vi "Custom Automation Tool.vi"(8 "error in (no error)":errorcluster) -> (0 "error out":errorcluster)   [LabVIEW 2021]
doc: "Presents an interface to either update a specification limit, or add a new one."
uses:
  CTLs/Step.ctl
  CTLs/Step Type.ctl
  <vilib>/Utility/config.llb/Config Data RefNum.ctl
  <vilib>/Utility/miscctls.llb/LVRowAndColumnUnsignedTypeDef.ctl
  CTLs/FGV Actions.ctl
  bd503c13-d10c-440e-ab5e-4e60baef5deb.vi
  cc7d3372-ed48-481f-8659-91fce09351ce.vi
  <vilib>/Utility/config.llb/Write Key (String).vi
  <vilib>/Utility/config.llb/Read Key (String).vi
  <userlib>/_MGI/Application Control/MGI Gray if/MGI Gray if False.vi
  <vilib>/Utility/inputDevices.llb/closeKeyboard.vi
  <vilib>/Utility/inputDevices.llb/keyboardAcquire.vi
  <vilib>/Utility/config.llb/NI_LVConfig.lvlib
  FaKI State Machine/FaKI State Machine.lvlib
panel:
  in  "Export":bool
  in  "Import":bool
  out "Application Hotkey":string
  in  "Delete":bool
  in  "Start/Stop":bool
  in  "N":i32 caption="Times to Repeat\n(-1 = indefinitely)" min=-1
  in  "Activation Type":enum32{"Hotkey", "Automatic"}(radio)
  out "Menu":bool
  out "Row":i32
  in  "Add Step 2":bool
  in  "Dbl Click":T1
  out "Table":string[][](table)
  in  "Clear Profile":bool
  in  "Delete Step":bool
  in  "Insert Step":bool
  in  "Add Step":bool
  in  "Modify Step":bool
  in  "Close":bool
  in  "Save":bool
  in  "Restore":bool
  in  "Help":bool
  in  "Process Name":string(combo)
  # "Table has double-click\nfunctionality"
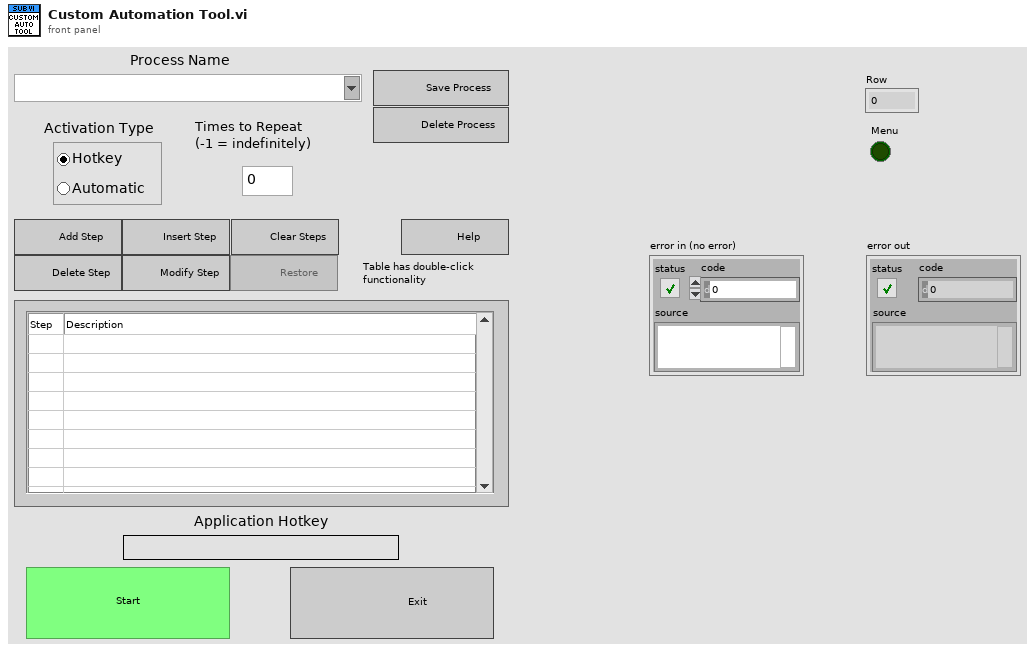
[diagram p1: front panel]
types:
  T1 = cluster{"Insert Before":bool, "Insert After":bool, "Modify":bool, "Delete":bool}
  T2 = enum8{"Enabled", "Disabled", "Disabled and Grayed Out"}
  T3 = typedef "LVPoint32TypeDef.ctl" = cluster{"Horizontal":i32, "Vertical":i32}
  T4 = typedef "LVRowAndColumnTypeDef.ctl" = cluster{"Row":i32, "Column":i32}
  T5 = enum32{"Invalid", "Standard", "Closed", "Hidden", "Minimized", "Maximized"}
  T6 = enum32{"invalid app kind", "Development System", "Run Time System", "Student Edition", "Embedded LabVIEW", "Evaluation", "Custom"}
  T7 = typedef "Step.ctl" = cluster{"Type":T8, "Coords":cluster{"x":i32, "y":i32}, "Delay":i32, "Key":u8, "Repeat":i32, "RClick?":bool}
  T8 = typedef "Step Type.ctl" = enum16{"Mouse Move", "Mouse Click", "Key Press", "Wait", "Mouse Down", "Mouse Up", "Key Down", "Key Up"}
  T9 = typedef "LVRowAndColumnUnsignedTypeDef.ctl" = cluster{"Row":u32, "Column":u32}
  T10 = cluster{"Steps":T7[], "Activation Type":enum32{"Hotkey", "Automatic"}, "N":i32}
  T11 = typedef "FGV Actions.ctl" = enum16{"Read", "Write"}
  T12 = typedef "NI_LVConfig.lvlib/Config Data RefNum.ctl" = refnum<k1>
  T13 = cluster{"Core":cluster{"Current VI Reference":refnum<vi>, "Close Panel on Exit?":bool}, "Steps":T7[], "Refs":refnum<vi>[], "Config":T12, "Step":i32, "n":i32, "Hotkey":enum16{"0", "1", "2", "3", "4", "5", "6", "7", "8", "9", "A", "B", "C", "D", "E", "F", "G", "H", "I", "J", "K", "L", "M", "N", "O", "P", "Q", "R", "S", "T", "U", "V", "W", "X", "Y", "Z", "F1", "F2", "F3", "F4", "F5", "F6", "F7", "F8", "F9", "F10", "F11", "F12", "F13", "F14", "F15", "ADD", "BACK", "BACKSLASH", "CAPITAL", "COMMA", "DECIMAL", "DELETE", "DIVIDE", "DOWN", "END", "EQUALS", "ESCAPE", "GRAVE (`)", "HOME", "INSERT", "LBRACKET", "LCONTROL", "LEFT", "L ALT", "LSHIFT", "LWIN", "MINUS", "MULTIPLY", "NEXT", "NUMLOCK", "NUMPAD_0", "NUMPAD_1", "NUMPAD_2", "NUMPAD_3", "NUMPAD_4", "NUMPAD_5", "NUMPAD_6", "NUMPAD_7", "NUMPAD_8", "NUMPAD_9", "PAUSE", "PERIOD", "PRIOR (PG UP)", "RBRACKET", "RCONTROL", "RETURN", "RIGHT", "R ALT", "RSHIFT", "RWIN", "SCROLL", "SEMICOLON", "SLASH", "SPACE", "SUBTRACT", "TAB", "UP", "ENTER (num pad)", "' (quote)"}[], "Keyboard":refnum<k1>}
  T14 = enum16{"0", "1", "2", "3", "4", "5", "6", "7", "8", "9", "A", "B", "C", "D", "E", "F", "G", "H", "I", "J", "K", "L", "M", "N", "O", "P", "Q", "R", "S", "T", "U", "V", "W", "X", "Y", "Z", "F1", "F2", "F3", "F4", "F5", "F6", "F7", "F8", "F9", "F10", "F11", "F12", "F13", "F14", "F15", "ADD", "BACK", "BACKSLASH", "CAPITAL", "COMMA", "DECIMAL", "DELETE", "DIVIDE", "DOWN", "END", "EQUALS", "ESCAPE", "GRAVE (`)", "HOME", "INSERT", "LBRACKET", "LCONTROL", "LEFT", "L ALT", "LSHIFT", "LWIN", "MINUS", "MULTIPLY", "NEXT", "NUMLOCK", "NUMPAD_0", "NUMPAD_1", "NUMPAD_2", "NUMPAD_3", "NUMPAD_4", "NUMPAD_5", "NUMPAD_6", "NUMPAD_7", "NUMPAD_8", "NUMPAD_9", "PAUSE", "PERIOD", "PRIOR (PG UP)", "RBRACKET", "RCONTROL", "RETURN", "RIGHT", "R ALT", "RSHIFT", "RWIN", "SCROLL", "SEMICOLON", "SLASH", "SPACE", "SUBTRACT", "TAB", "UP", "ENTER (num pad)", "' (quote)"}[]
  T15 = cluster{"Current VI Reference":refnum<vi>, "Close Panel on Exit?":bool}
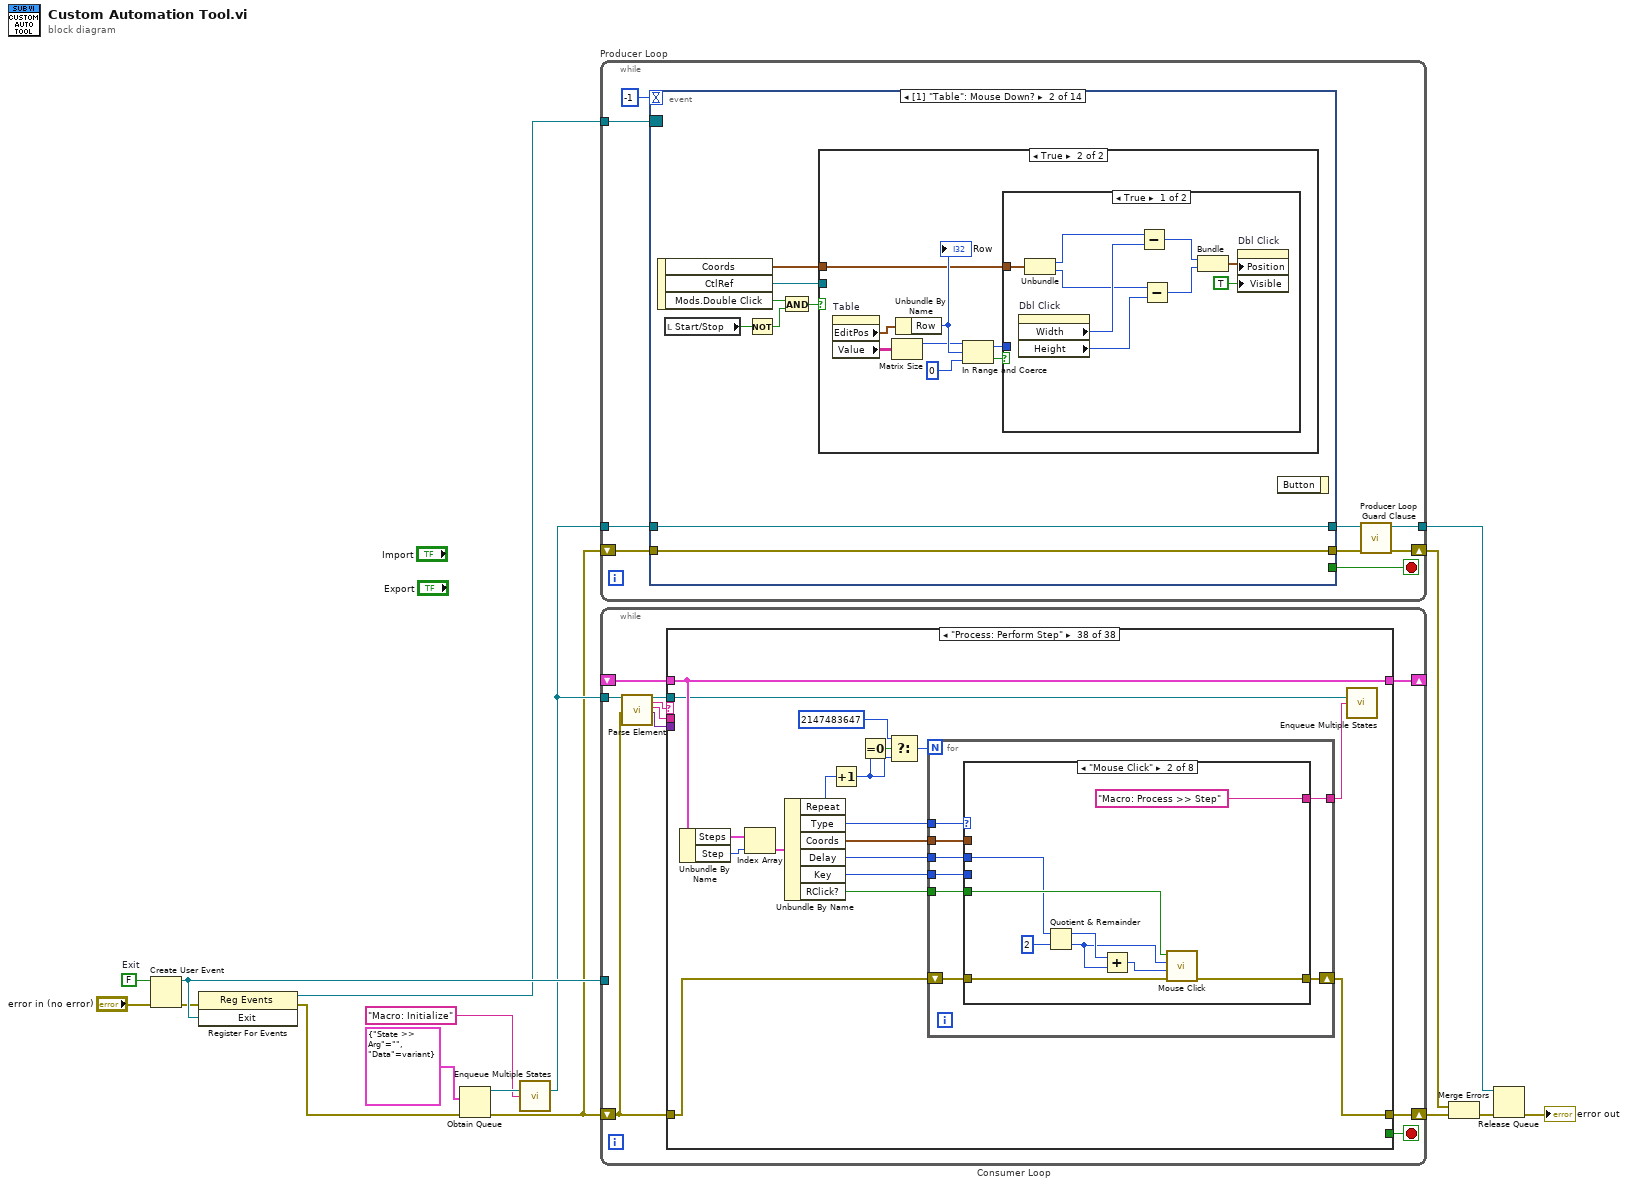
[diagram p0: block diagram]
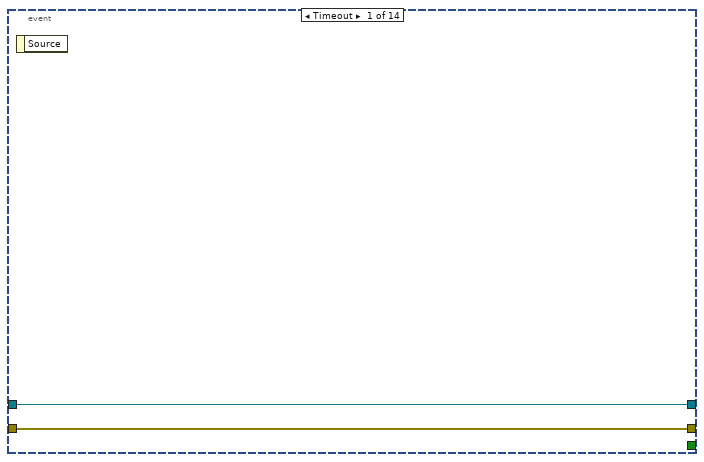
[diagram p2: hidden frame]
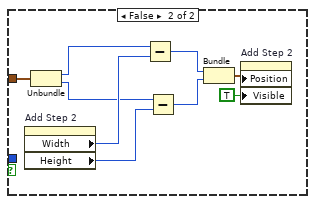
[diagram p4: hidden frame]
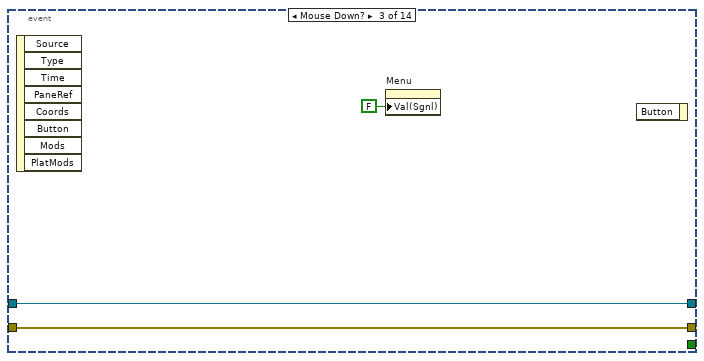
[diagram p5: hidden frame]
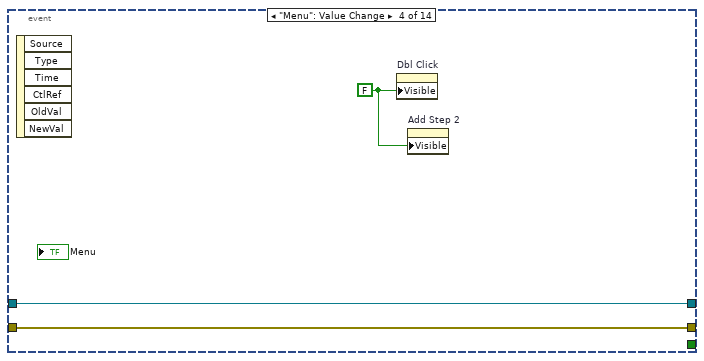
[diagram p6: hidden frame]
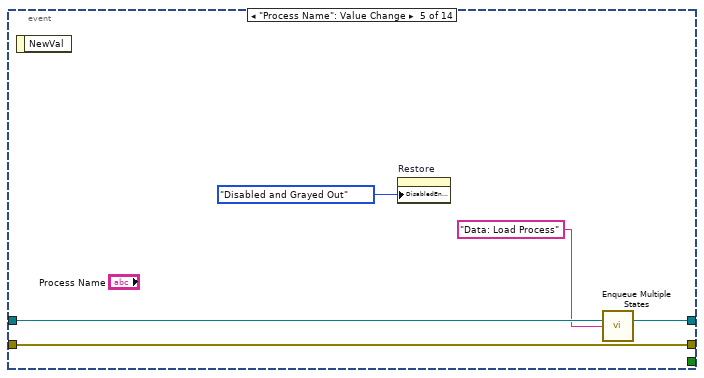
[diagram p7: hidden frame]
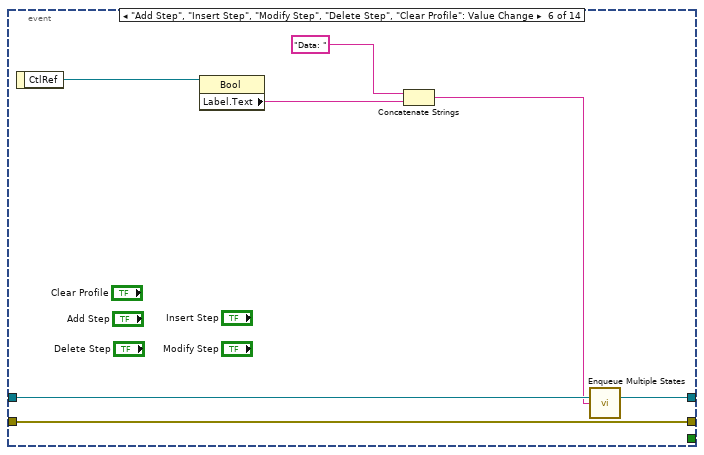
[diagram p8: hidden frame]
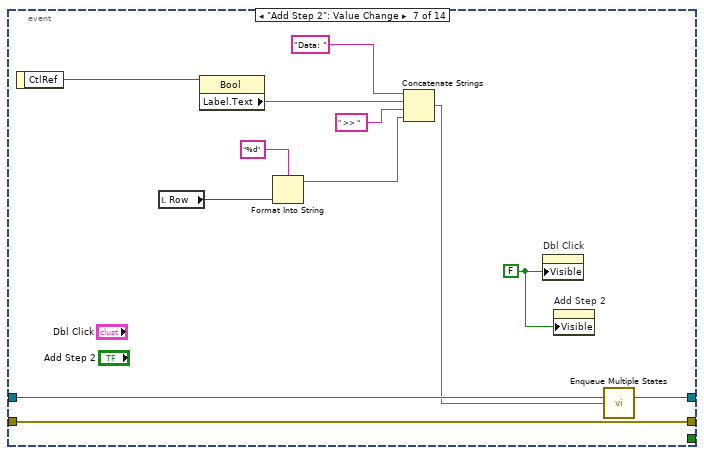
[diagram p9: hidden frame]
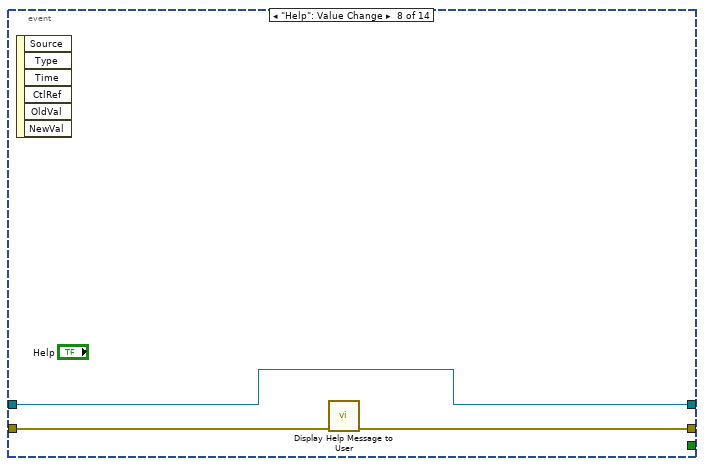
[diagram p10: hidden frame]
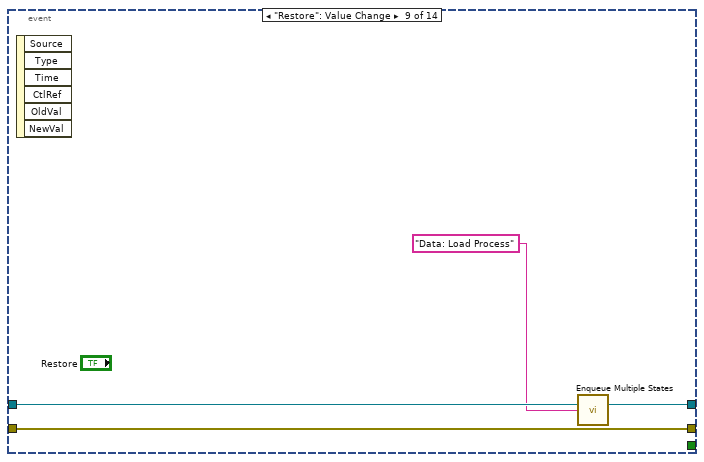
[diagram p11: hidden frame]
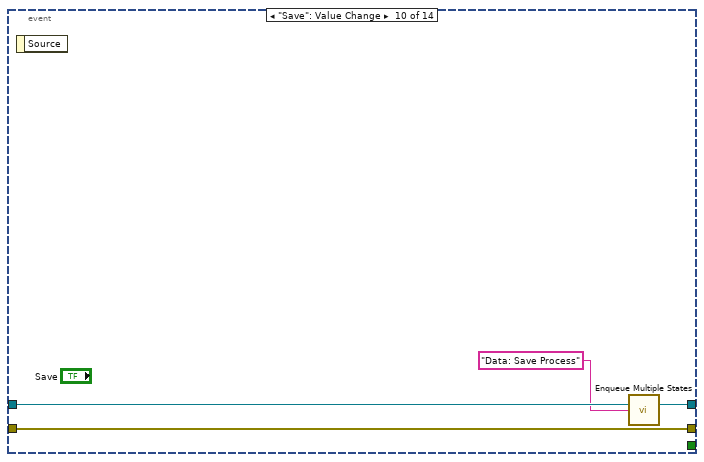
[diagram p12: hidden frame]
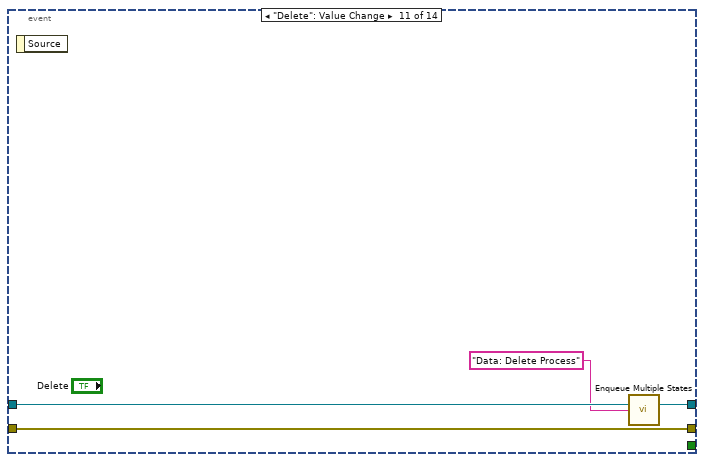
[diagram p13: hidden frame]
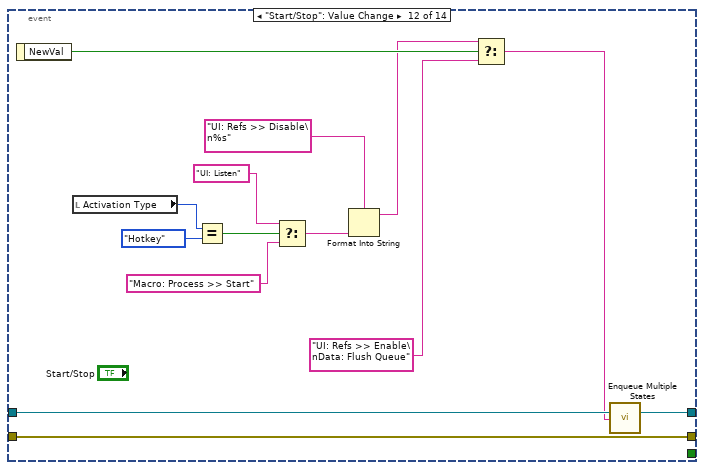
[diagram p14: hidden frame]
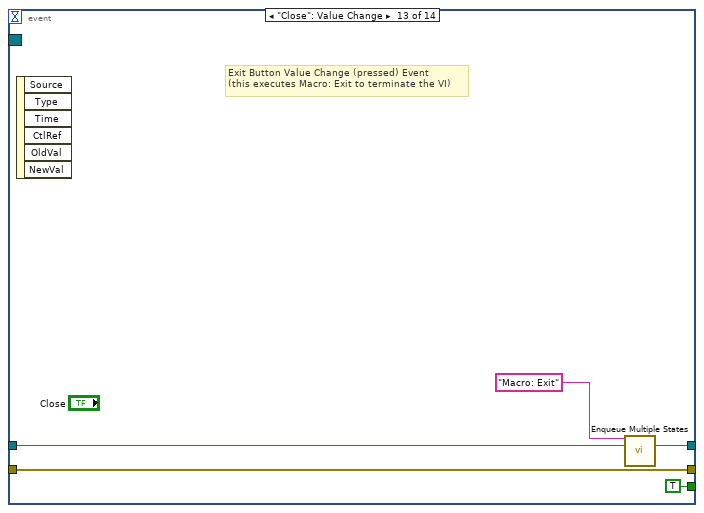
[diagram p15: hidden frame]
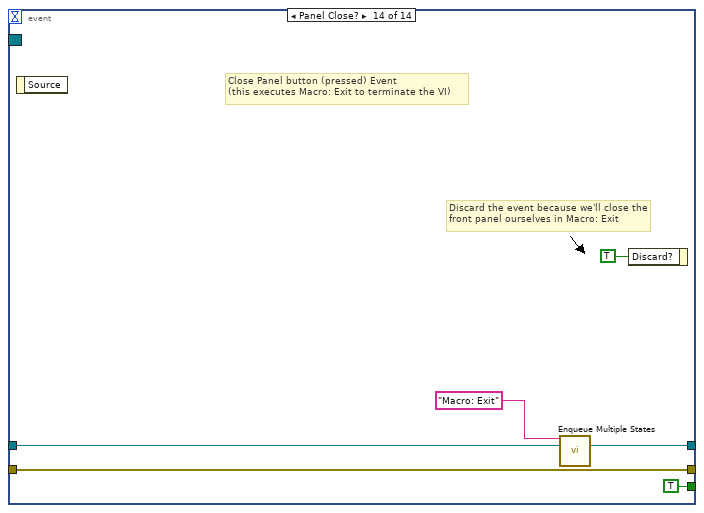
[diagram p16: hidden frame]
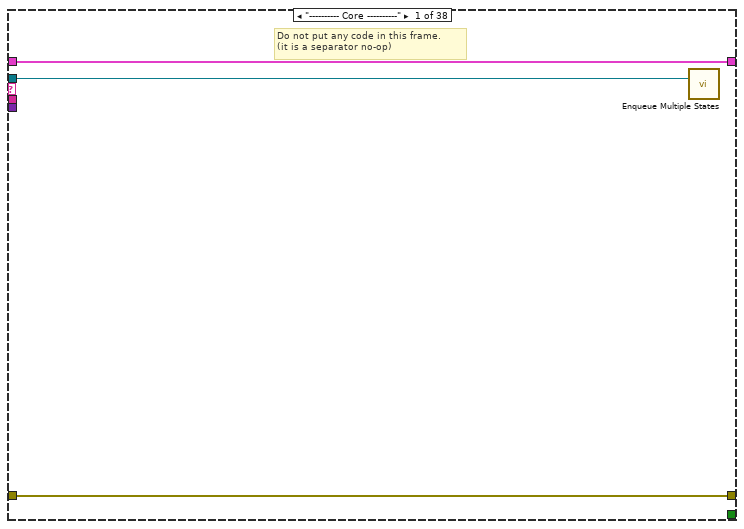
[diagram p17: hidden frame]
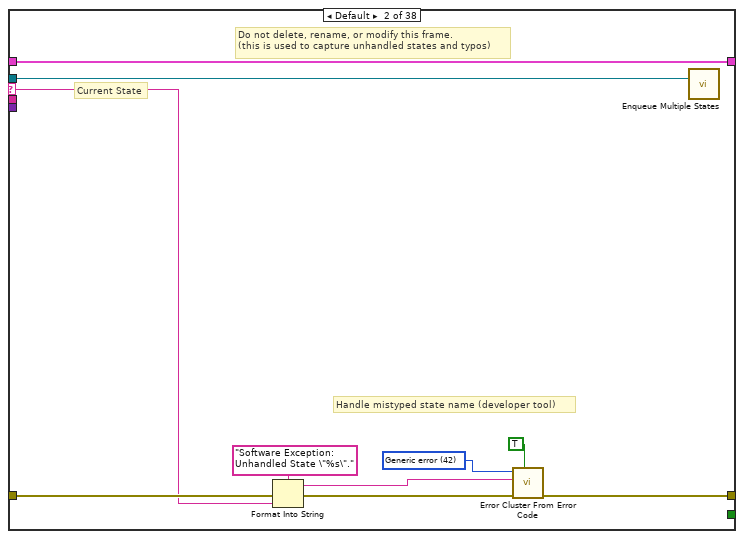
[diagram p18: hidden frame]
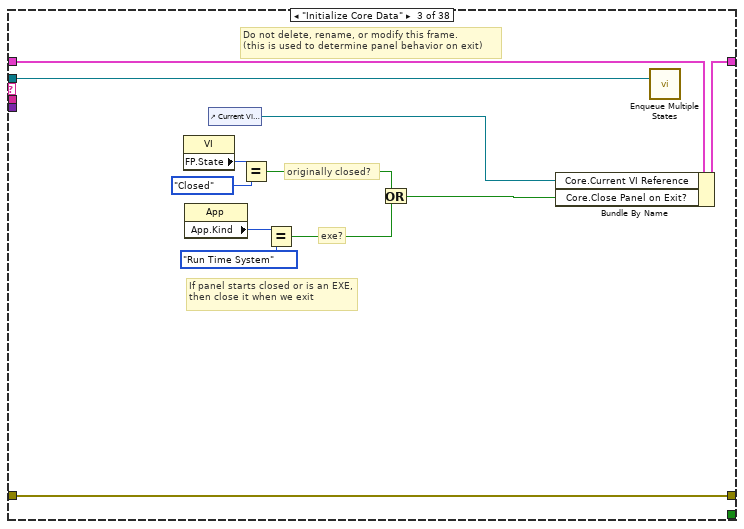
[diagram p19: hidden frame]
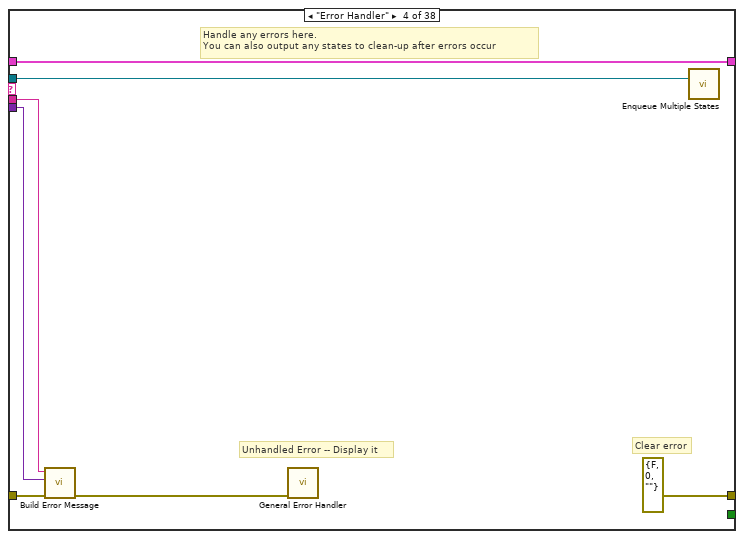
[diagram p20: hidden frame]
diagram:
  w13 = FALSE  # Exit
  n1 = Create User Event(user event datatype=w13, error in="error in (no error)") -> (user event=w16:refnum<user-event>, error out=w12:errorcluster)
  n2 = register-events(error in=w12, w16) -> (reference out=w15:refnum<event-registration>, error out=w14:errorcluster)  [unwired: 1 in]
  n3 = Obtain Queue(element data type=cluster{"State >> Arg":string, "Data":variant} {"State >> Arg"="", "Data"=variant}, error in (no error)=w14) -> (queue out=w6:refnum<queue>, error out=w3:errorcluster)  [unwired: 3 in, 1 out]
  n4 = call "Enqueue Multiple States.vi"("queue in"=w6, "State(s) at Back"="Macro: Initialize") -> ("queue out"=w7:refnum<queue>)  [unwired: 13 in]
  n5 = while "Producer Loop" {
    shift-right: [w25] -> w9
    shift-left: w3 -> [w23]
    tunnel: w15 -> [w19]
    tunnel: w7 -> [w21]
    tunnel: [w24] -> w11
    stop <- w18 stop-if-true
    n6 = event shown="[1] \"Table\": Mouse Down?" {
      selector: w19 -> [_ _ _ _ _ _ _ _ _ _ _ _ _ _]
      dyn-events: _ -> [_ _ _ _ _ _ _ _ _ _ _ _ _ _]
      timeout: -1 ("Timeout") -> [_ _ _ _ _ _ _ _ _ _ _ _ _ _]
      tunnel: [w27 w35 w64 w67 w72 w79 w91 w93 w98 w102 w106 w120 w125 w131] -> w22
      tunnel: w23 -> [w27 w35 w64 w67 w72 w79 w91 w94 w98 w102 w106 w120 w125 w131]
      tunnel: w21 -> [w26 w32 w62 w65 w70 w75 w82 w92 w96 w101 w105 w108 w123 w128]
      tunnel: [w26 w32 w62 w65 w69 w74 w81 w92 w97 w100 w104 w109 w122 w127] -> w20
      tunnel: [_ _ _ _ _ _ _ _ _ _ _ _ TRUE TRUE] -> w18
      event Timeout {
        n7 = event-data() -> ()  [unwired: 1 in, 1 out]
      }
      event "Table": Mouse Down? {
        n8 = event-data() -> ("Coords"=w33:T3, "CtlRef"=w34:refnum<vi>, "Mods.Double Click"=w29:bool)  [unwired: 1 in]
        n9 = local read "Start/Stop"() -> (w31:bool)
        n10 = Not(x=w31) -> (.not. x?=w30:bool)
        n11 = And(x=w29, y=w30) -> (x .and. y?=w28:bool)
        n12 = case shown="True" w28 {
          tunnel: w34 -> [_ _]
          tunnel: w33 -> [_ w36]
          frame False {
          }
          frame True {
            n13 = property on="Table" class="Tbl (strict)"() -> ("EditPos"=w42:T4, "Value"=w43:string[][])  [unwired: 2 in, 2 out]
            n14 = Matrix Size(0:w43) -> (1:w40:i32)  [unwired: 1 out]
            n15 = Unbundle By Name(w42) -> ("Row"=w41:i32)
            "Row" <- w41
            n16 = In Range and Coerce(upper limit=w40, x=w41, lower limit=0) -> (coerced(x)=w37:i32, In Range?=w38:bool)
            n17 = case shown="True" w38 {
              tunnel: w37 -> [_ _]
              tunnel: w36 -> [w51 w60]
              frame True {
                n18 = property on="Dbl Click" class="Clust"() -> ("Width"=w49:u32, "Height"=w48:u32)  [unwired: 2 in, 2 out]
                n19 = Unbundle(w51) -> ("Horizontal"=w50:i32, "Vertical"=w47:i32)
                n20 = Subtract(x=w50, y=w49) -> (x-y=w45:u32)
                n21 = Subtract(x=w47, y=w48) -> (x-y=w46:u32)
                n22 = Bundle(w45, w46) -> (w44:cluster{u32, u32})  [unwired: 1 in]
                n23 = property on="Dbl Click" class="Clust"("Position"=w44, "Visible"=TRUE) -> ()  [unwired: 2 in, 2 out]
              }
              frame False {
                n24 = property on="Add Step 2" class="Bool"() -> ("Width"=w58:u32, "Height"=w57:u32)  [unwired: 2 in, 2 out]
                n25 = Unbundle(w60) -> ("Horizontal"=w59:i32, "Vertical"=w56:i32)
                n26 = Subtract(x=w59, y=w58) -> (x-y=w54:u32)
                n27 = Subtract(x=w56, y=w57) -> (x-y=w55:u32)
                n28 = Bundle(w54, w55) -> (w53:cluster{u32, u32})  [unwired: 1 in]
                n29 = property on="Add Step 2" class="Bool"("Position"=w53, "Visible"=TRUE) -> ()  [unwired: 2 in, 2 out]
              }
            }
          }
        }
        n30 = event-data() -> ()  [unwired: 2 in, 1 out]
      }
      event Mouse Down? {
        n31 = event-data() -> ()  [unwired: 1 in, 8 out]
        n32 = property on="Menu" class="Bool (strict)"("Val(Sgnl)"=FALSE ("Value (Signaling)")) -> ()  [unwired: 2 in, 2 out]
        n33 = event-data() -> ()  [unwired: 2 in, 1 out]
      }
      event "Menu": Value Change {
        w66 = FALSE ("Visible")
        n34 = event-data() -> ()  [unwired: 1 in, 6 out]
        n35 = property on="Dbl Click" class="Clust"("Visible"=w66) -> ()  [unwired: 2 in, 2 out]
        n36 = property on="Add Step 2" class="Bool"("Visible"=w66) -> ()  [unwired: 2 in, 2 out]
      }
      event "Process Name": Value Change {
        n37 = event-data() -> ()  [unwired: 1 in, 1 out]
        n38 = property on="Restore" class="Bool"("DisabledEnum"=T2."Disabled and Grayed Out" ("Disabled")) -> ()  [unwired: 2 in, 2 out]
        n39 = call "Enqueue Multiple States.vi"("queue in"=w70, "State(s) at Back"="Data: Load Process" ("string")) -> ("queue out"=w69:refnum<queue>)  [unwired: 13 in]
      }
      event "Add Step", "Insert Step", "Modify Step", "Delete Step", "Clear Profile": Value Change {
        n40 = event-data() -> ("CtlRef"=w78:refnum<vi>)  [unwired: 1 in]
        n41 = property class="Bool"(reference=w78) -> ("Label.Text"=w76:string)  [unwired: 1 in, 2 out]
        n42 = Concatenate Strings("Data: " ("State(s) at Back (\"\")"), w76) -> (w73:string)
        n43 = call "Enqueue Multiple States.vi"("queue in"=w75, "State(s) at Back"=w73) -> ("queue out"=w74:refnum<queue>)  [unwired: 13 in]
      }
      event "Dbl Click.Insert Before", "Dbl Click.Insert After", "Dbl Click.Modify", "Dbl Click.Delete", "Add Step 2": Value Change {
        w84 = FALSE ("Visible")
        n44 = event-data() -> ("CtlRef"=w90:refnum<vi>)  [unwired: 1 in]
        n45 = local read "Row"() -> (w83:i32)
        n46 = property class="Bool"(reference=w90) -> ("Label.Text"=w88:string)  [unwired: 1 in, 2 out]
        n47 = Format Into String(format string="%d", w83) -> (resulting string=w85:string)  [unwired: 2 in, 1 out]
        n48 = Concatenate Strings("Data: " ("State(s) at Back (\"\")"), w88, " >> " ("string"), w85) -> (w80:string)
        n49 = property on="Dbl Click" class="Clust"("Visible"=w84) -> ()  [unwired: 2 in, 2 out]
        n50 = property on="Add Step 2" class="Bool"("Visible"=w84) -> ()  [unwired: 2 in, 2 out]
        n51 = call "Enqueue Multiple States.vi"("queue in"=w82, "State(s) at Back"=w80) -> ("queue out"=w81:refnum<queue>)  [unwired: 13 in]
      }
      event "Help": Value Change {
        n52 = event-data() -> ()  [unwired: 1 in, 6 out]
        n53 = call "Display Help Message to User"("error in (no error)"=w94) -> ("error out"=w93:errorcluster)  [unwired: 9 in, 1 out]
      }
      event "Restore": Value Change {
        n54 = event-data() -> ()  [unwired: 1 in, 6 out]
        n55 = call "Enqueue Multiple States.vi"("queue in"=w96, "State(s) at Back"="Data: Load Process" ("State(s) at Back (\"\")")) -> ("queue out"=w97:refnum<queue>)  [unwired: 13 in]
      }
      event "Save": Value Change {
        n56 = event-data() -> ()  [unwired: 1 in, 1 out]
        n57 = call "Enqueue Multiple States.vi"("queue in"=w101, "State(s) at Back"="Data: Save Process" ("State(s) at Back (\"\")")) -> ("queue out"=w100:refnum<queue>)  [unwired: 13 in]
      }
      event "Delete": Value Change {
        n58 = event-data() -> ()  [unwired: 1 in, 1 out]
        n59 = call "Enqueue Multiple States.vi"("queue in"=w105, "State(s) at Back"="Data: Delete Process" ("State(s) at Back (\"\")")) -> ("queue out"=w104:refnum<queue>)  [unwired: 13 in]
      }
      event "Start/Stop": Value Change {
        n60 = event-data() -> ("NewVal"=w112:bool)  [unwired: 1 in]
        n61 = local read "Activation Type"() -> (w119:enum32{"Hotkey", "Automatic"})
        n62 = Equal?(x=w119, y=enum32{"Hotkey", "Automatic"}."Hotkey") -> (x = y?=w117:bool)
        n63 = Select(t="UI: Listen", s=w117, f="Macro: Process >> Start") -> (s? t:f=w114:string)
        n64 = Format Into String(format string="UI: Refs >> Disable\n%s" ("State(s) at Back (\"\")"), w114) -> (resulting string=w111:string)  [unwired: 2 in, 1 out]
        n65 = Select(t=w111, s=w112, f="UI: Refs >> Enable\nData: Flush Queue") -> (s? t:f=w107:string)
        n66 = call "Enqueue Multiple States.vi"("queue in"=w108, "State(s) at Back"=w107) -> ("queue out"=w109:refnum<queue>)  [unwired: 13 in]
      }
      event "Close": Value Change {
        # "Exit Button Value Change (pressed) Event\n(this executes Macro: Exit to terminate the VI)"
        n67 = event-data() -> ()  [unwired: 1 in, 6 out]
        n68 = call "Enqueue Multiple States.vi"("State(s) at Front"="Macro: Exit", "queue in"=w123) -> ("queue out"=w122:refnum<queue>)  [unwired: 13 in]
      }
      event Panel Close? {
        # "Discard the event because we'll close the front panel ourselves in Macro: Exit"
        # "Close Panel button (pressed) Event\n(this executes Macro: Exit to terminate the VI)"
        n69 = event-data() -> ()  [unwired: 1 in, 1 out]
        n70 = call "Enqueue Multiple States.vi"("State(s) at Front"="Macro: Exit", "queue in"=w128) -> ("queue out"=w127:refnum<queue>)  [unwired: 13 in]
        n71 = event-data("Discard?"=TRUE) -> ()  [unwired: 1 in, 1 out]
      }
    }
    n72 = call "Producer Loop Guard Clause.vi"("error in (no error)"=w22, "queue in"=w20) -> ("error out"=w25:errorcluster, "queue out"=w24:refnum<queue>)  [unwired: 8 in]
  }
  n73 = while "Consumer Loop" {
    shift-right: [w136] -> _
    shift-left: _ -> [w137]
    shift-right: [w139] -> w8
    shift-left: w3 -> [w140]
    tunnel: w7 -> [w141]
    tunnel: w16 -> [_]
    stop <- w138 stop-if-true
    n74 = call "Parse Element.vi"("queue in"=w141, "error in (no error)"=w140) -> ("queue out"=w135:refnum<queue>, "State"=w134:string, "Arg"=w133:string, "Data"=w132:variant)  [unwired: 14 in]
    n75 = case shown="\"Process: Perform Step\"" w134 {
      selector: w134 -> [_ w146 _ _ _ _ _ _ _ _ _ _ _ _ _ _ _ _ _ _ _ _ _ _ _ _ _ _ _ _ _ _ _ _ _ _ _ _]
      tunnel: w135 -> [w142 w145 w155 w167 w174 w178 w184 w207 _ w217 w225 w233 w241 w249 w257 w268 w280 w291 w302 _ w354 _ w396 w401 w410 w412 w421 _ w497 _ w522 w532 w545 w548 w553 w597 w604 w608]
      tunnel: w133 -> [_ _ _ w169 _ _ _ _ _ _ _ _ _ _ w259 w271 w282 w293 _ _ _ _ _ _ _ w413 w422 _ _ w515 _ _ _ _ w556 _ _ _]
      tunnel: w137 -> [w143 w148 w161 w172 w177 w179 _ w208 w212 w220 w226 w234 w242 w250 w260 w272 w283 w294 w304 w314 w351 w380 w400 w402 w406 w416 w424 w496 w510 w514 w530 w535 w546 w550 w552 w602 w605 w624]
      tunnel: [w144 w150 w165 errorcluster {"status"=FALSE, "code"=0, "source"=""} ("error out") w176 w180 w186 w209 w213 w221 w229 w237 w245 w253 w263 w275 w286 w297 w307 w321 w360 w381 w398 w403 w408 w414 w425 w494 w507 w513 w529 w536 w547 w551 w557 w603 w606 w615] -> w139
      tunnel: w140 -> [w144 w149 w165 w171 w176 w180 w187 w209 w214 w221 w229 w237 w245 w253 w263 w275 w286 w297 w307 w323 w365 w382 w397 w403 w409 w415 w426 w495 w508 w513 w526 w537 w547 w551 w557 w603 w606 w616]
      tunnel: [_ _ _ _ TRUE _ _ _ _ _ _ _ _ _ _ _ _ _ _ _ _ _ _ _ _ _ _ _ _ _ _ _ _ _ _ _ _ _] -> w138
      tunnel: [w143 w148 w166 w172 w177 w179 w206 w208 w211 w219 w228 w236 w244 w252 w262 w274 w285 w296 w303 w320 w352 w380 w400 w402 w405 w416 w424 w496 w510 w514 w530 w535 w546 w550 w555 w602 w605 w624] -> w136
      tunnel: w132 -> [_ _ _ w168 _ _ _ _ _ _ _ _ _ _ _ _ _ _ _ _ _ _ _ _ _ _ _ _ _ _ _ _ _ _ _ _ _ _]
      frame "---------- Core ----------" {
        # "Do not put any code in this frame.\n(it is a separator no-op)"
        n76 = call "Enqueue Multiple States.vi"("queue in"=w142) -> ()  [unwired: 14 in, 1 out]
      }
      frame Default {
        w153 = 42 items=["No error", "Argument error", "Memory is full", "Out of zone", "End of file", "File already open", "Generic file I/O error", "File not found", "File permission error", "Disk is full", "Duplicate path", "Too many files open", "System feature not enabled", "Resource file not found", "Cannot add resource", "Resource not found", "Image not found", "Image memory error", "Pen does not exist", "Config type invalid", "Config token not found", "Config parse error", "Config memory error", "Bad external code format", "Bad external code offset", "External code not present", "Null window", "Destroy window error", "Null menu", "Print aborted", "Bad print record", "Print driver error", "Windows error during printing", "Memory error during printing", "Print dialog error", "Generic print error", "Invalid device refnum", "Device not found", "Device parameter error", "Device unit error", "Cannot open device", "Device call aborted", "Generic error", "Cancelled by user", "Object ID too low", "Object ID too high", "Object not in heap", "Unknown heap", "Unknown object (invalid DefProc)", "Unknown object (DefProc not in table)", "Message out of range", "Invalid (null) method", "Unknown message", "Manager call not supported", "Bad address", "Network operation in progress", "Network operation timed out", "Connection is busy", "Network attribute not supported", "Network error", "Address in use", "System out of memory", "Connection aborted", "Connection refused", "Not connected", "Already connected", "Connection closed", "Initialization error (interapplication manager)", "Bad occurrence", "Wait on unbound occurrence handler", "Occurrence queue overflow", "Datalog type conflict", "Unused", "Unrecognized type (interapplication manager)", "Memory corrupt", "Failed to make temporary DLL", "Old CIN version", "Drag socket not found", "Failed to load drop-object", "Failed to register OLE object", "Failed to release OLE object", "Format specifier type mismatch", "Unknown format specifier", "Too few format specifiers", "Too many format specifiers", "Scan failed", "Newer CIN version", "Error converting to variant", "Runtime menu error", "Password tampered", "Variant attribute not found", "Incompatible variant data type", "Event data is not available", "Event Store is not present", "Occurrence is not found", "Event Queue is not created", "Event info is not available", "Refnum passed is NULL", "Error retrieving Class GUID", "Error retrieving CoClass GUID", "Error retrieving TypeLib GUID.", "Bad built application magic bytes.", "Specific driver is different from the specific driver associated with the Logical Name.", "There is no session opened to the class driver.", "Max Error", "MAX - Error with config objects", "MAX - Error loading configuration", "MAX - Group not supported"]
        # "Current State"
        # "Do not delete, rename, or modify this frame.\n(this is used to capture unhandled states and typos)"
        # "Handle mistyped state name (developer tool)"
        n77 = Format Into String(format string="Software Exception: Unhandled State \"%s\"." ("message"), error in=w149, w146) -> (resulting string=w152:string, error out=w151:errorcluster)  [unwired: 1 in]
        n78 = call <vilib>:"Error Cluster From Error Code.vi"("show call chain? (False)"=TRUE, "error in (no error)"=w151, "error message (\"\")"=w152, "error code (0)"=w153) -> ("error out"=w150:errorcluster)  [unwired: 5 in]
        n79 = call "Enqueue Multiple States.vi"("queue in"=w145) -> ()  [unwired: 14 in, 1 out]
      }
      frame "Initialize Core Data" {
        # "Do not delete, rename, or modify this frame.\n(this is used to determine panel behavior on exit)"
        # "originally closed?"
        # "exe?"
        # "If panel starts closed or is an EXE, then close it when we exit"
        n80 = property class="VI"() -> ("FP.State"=w158:T5)  [unwired: 2 in, 2 out]
        n81 = property class="App"() -> ("App.Kind"=w164:T6)  [unwired: 2 in, 2 out]
        n82 = control-ref of="Current VI Reference"() -> (w159:refnum<vi>)
        n83 = Equal?(x=w158, y=T5."Closed" ("Front Panel Window:State")) -> (x = y?=w156:bool)
        n84 = Equal?(x=w164, y=T6."Run Time System" ("Application:Kind")) -> (x = y?=w162:bool)
        n85 = Or(x=w156, y=w162) -> (x .or. y?=w160:bool)
        n86 = Bundle By Name(cluster=w161, "Core.Current VI Reference"=w159, "Core.Close Panel on Exit?"=w160) -> (w166:T13)
        n87 = call "Enqueue Multiple States.vi"("queue in"=w155) -> ()  [unwired: 14 in, 1 out]
      }
      frame "Error Handler" {
        # "Unhandled Error -- Display it"
        # "Handle any errors here.\nYou can also output any states to clean-up after errors occur"
        # "Clear error"
        n88 = call "Build Error Message.vi"("error in (no error)"=w171, "Data"=w168, "Arg"=w169) -> ("error out"=w170:errorcluster)  [unwired: 8 in]
        n89 = call <vilib>:"General Error Handler.vi"("error in (no error)"=w170) -> ()  [unwired: 10 in, 5 out]
        n90 = call "Enqueue Multiple States.vi"("queue in"=w167) -> ()  [unwired: 14 in, 1 out]
      }
      frame "Exit" {
        # "Do not put any code in this frame.\n(No errors that occur here will be handled.)"
        n91 = call "Enqueue Multiple States.vi"("queue in"=w174) -> ()  [unwired: 14 in, 1 out]
      }
      frame "---------- Data ----------" {
        # "Do not put any code in this frame.\n(It is a separator no-op. You can make a copy of this frame to create a new Data frame)"
        n92 = call "Enqueue Multiple States.vi"("queue in"=w178) -> ()  [unwired: 14 in, 1 out]
      }
      frame "Data: Initialize" {
        w182 = T14 [] items=["0", "1", "2", "3", "4", "5", "6", "7", "8", "9", "A", "B", "C", "D", "E", "F", "G", "H", "I", "J", "K", "L", "M", "N", "O", "P", "Q", "R", "S", "T", "U", "V", "W", "X", "Y", "Z", "F1", "F2", "F3", "F4", "F5", "F6", "F7", "F8", "F9", "F10", "F11", "F12", "F13", "F14", "F15", "ADD", "BACK", "BACKSLASH", "CAPITAL", "COMMA", "DECIMAL", "DELETE", "DIVIDE", "DOWN", "END", "EQUALS", "ESCAPE", "GRAVE (`)", "HOME", "INSERT", "LBRACKET", "LCONTROL", "LEFT", "L ALT", "LSHIFT", "LWIN", "MINUS", "MULTIPLY", "NEXT", "NUMLOCK", "NUMPAD_0", "NUMPAD_1", "NUMPAD_2", "NUMPAD_3", "NUMPAD_4", "NUMPAD_5", "NUMPAD_6", "NUMPAD_7", "NUMPAD_8", "NUMPAD_9", "PAUSE", "PERIOD", "PRIOR (PG UP)", "RBRACKET", "RCONTROL", "RETURN", "RIGHT", "R ALT", "RSHIFT", "RWIN", "SCROLL", "SEMICOLON", "SLASH", "SPACE", "SUBTRACT", "TAB", "UP", "ENTER (num pad)", "' (quote)"]  # Hotkey
        w185 = refnum<k1> refnum items=["KEYBOARD"]  # Keyboard
        w189 = 0  # n
        w190 = 0  # Step
        w194 = T12 refnum items=["config data"]  # Config
        w195 = T7[] []  # Steps
        w199 = refnum<vi>[] []  # Refs
        w205 = T15 {"Current VI Reference"=refnum, "Close Panel on Exit?"=FALSE}  # Core
        # "Initialize the shift-register data, here.\n(data names are defined by what you wire into the bundle function)"
        n93 = control-ref of="Activation Type"() -> (w193:refnum<vi>)
        n94 = control-ref of="Process Name"() -> (w191:refnum<vi>)
        n95 = control-ref of="Add Step"() -> (w204:refnum<vi>)
        n96 = control-ref of="Delete Step"() -> (w202:refnum<vi>)
        n97 = control-ref of="Insert Step"() -> (w201:refnum<vi>)
        n98 = control-ref of="Modify Step"() -> (w203:refnum<vi>)
        n99 = control-ref of="Save"() -> (w200:refnum<vi>)
        n100 = control-ref of="Clear Profile"() -> (w196:refnum<vi>)
        n101 = control-ref of="Delete"() -> (w181:refnum<vi>)
        n102 = control-ref of="N"() -> (w192:refnum<vi>)
        n103 = call <vilib>:"Intialize Keyboard.vi"("error in (no error)"=w187) -> ("error out"=w186:errorcluster, "device ID"=w188:refnum<k1>)  [unwired: 9 in]
        n104 = Type Cast(type=w185, x=w188) -> (*(type *) &x=w183:refnum<k1>)
        n105 = Build Array(w204, w202, w201, w203, w200, w196, w193, w192, w191, w181) -> (w198:refnum<vi>[])
        n106 = Insert Into Array(array=w199, new element=w198) -> (w197:refnum<vi>[])  [unwired: 1 in]
        n107 = Bundle("Core"=w205, "Steps"=w195, "Refs"=w197, "Config"=w194, "Step"=w190, "n"=w189, "Hotkey"=w182, "Keyboard"=w183) -> (w206:T13)  [unwired: 1 in]
        n108 = call "Enqueue Multiple States.vi"("queue in"=w184) -> ()  [unwired: 14 in, 1 out]
      }
      frame "Data: Flush Queue" {
        n109 = Flush Queue(queue=w207) -> ()  [unwired: 1 in, 3 out]
      }
      frame "Data: Open Config" {
        n110 = call "Config Paths.vi"("error in (no error)"=w214) -> ("error out"=w216:errorcluster, "Process Config"=w210:path)  [unwired: 7 in, 2 out]
        n111 = call <vilib>:"Open Config Data.vi"("error in (no error)"=w216, "configuration file path"=w210) -> ("error out"=w213:errorcluster, "refnum"=w215:T12)  [unwired: 7 in, 1 out]
        n112 = Bundle By Name(cluster=w212, "Config"=w215) -> (w211:T13)
      }
      frame "Data: Add Step" {
        n113 = in-place {
          n114 = in-place-cluster #1(w220) -> ("Steps"=w224:T7[])
          n115 = call "Alter Motor Profile.vi"("Action"=enum16{"Add", "Insert", "Modify", "Delete"}."Add", "Steps in"=w224) -> ("Steps out"=w223:T7[])  [unwired: 9 in]
          n116 = in-place-cluster #1("Steps"=w223) -> (w219:T13)
        }
        n117 = call "Enqueue Multiple States.vi"("queue in"=w217, "State(s) at Back"="UI: Display Process" ("State(s) at Back (\"\")")) -> ()  [unwired: 13 in, 1 out]
      }
      frame "Data: Insert Step" {
        n118 = in-place {
          n119 = in-place-cluster #2(w226) -> ("Steps"=w232:T7[])
          n120 = call "Alter Motor Profile.vi"("Action"=enum16{"Add", "Insert", "Modify", "Delete"}."Insert", "Steps in"=w232) -> ("Steps out"=w231:T7[])  [unwired: 9 in]
          n121 = in-place-cluster #2("Steps"=w231) -> (w228:T13)
        }
        n122 = call "Enqueue Multiple States.vi"("queue in"=w225, "State(s) at Back"="UI: Display Process" ("State(s) at Back (\"\")")) -> ()  [unwired: 13 in, 1 out]
      }
      frame "Data: Modify Step" {
        n123 = in-place {
          n124 = in-place-cluster #3(w234) -> ("Steps"=w240:T7[])
          n125 = call "Alter Motor Profile.vi"("Action"=enum16{"Add", "Insert", "Modify", "Delete"}."Modify", "Steps in"=w240) -> ("Steps out"=w239:T7[])  [unwired: 9 in]
          n126 = in-place-cluster #3("Steps"=w239) -> (w236:T13)
        }
        n127 = call "Enqueue Multiple States.vi"("queue in"=w233, "State(s) at Back"="UI: Display Process" ("State(s) at Back (\"\")")) -> ()  [unwired: 13 in, 1 out]
      }
      frame "Data: Delete Step" {
        n128 = in-place {
          n129 = in-place-cluster #4(w242) -> ("Steps"=w248:T7[])
          n130 = call "Alter Motor Profile.vi"("Action"=enum16{"Add", "Insert", "Modify", "Delete"}."Delete", "Steps in"=w248) -> ("Steps out"=w247:T7[])  [unwired: 9 in]
          n131 = in-place-cluster #4("Steps"=w247) -> (w244:T13)
        }
        n132 = call "Enqueue Multiple States.vi"("queue in"=w241, "State(s) at Back"="UI: Display Process" ("State(s) at Back (\"\")")) -> ()  [unwired: 13 in, 1 out]
      }
      frame "Data: Add Step 2" {
        n133 = in-place {
          n134 = in-place-cluster #5(w250) -> ("Steps"=w256:T7[])
          n135 = call "Alter Motor Profile V2.vi"("Action"=enum16{"Add", "Insert", "Modify", "Delete"}."Add", "Steps in"=w256) -> ("Steps out"=w255:T7[])  [unwired: 9 in]
          n136 = in-place-cluster #5("Steps"=w255) -> (w252:T13)
        }
        n137 = call "Enqueue Multiple States.vi"("queue in"=w249, "State(s) at Back"="UI: Display Process" ("State(s) at Back (\"\")")) -> ()  [unwired: 13 in, 1 out]
      }
      frame "Data: Insert Before" {
        n138 = Decimal String To Number(string=w259) -> (number=w258:i32)  [unwired: 2 in, 1 out]
        n139 = in-place {
          in-place-border: w258 -> [w264]
          n140 = in-place-cluster #6(w260) -> ("Steps"=w267:T7[])
          n141 = call "Alter Motor Profile V2.vi"("Action"=enum16{"Add", "Insert", "Modify", "Delete"}."Insert", "Step"=w264, "Steps in"=w267) -> ("Steps out"=w266:T7[])  [unwired: 8 in]
          n142 = in-place-cluster #6("Steps"=w266) -> (w262:T13)
        }
        n143 = call "Enqueue Multiple States.vi"("queue in"=w257, "State(s) at Back"="UI: Display Process" ("State(s) at Back (\"\")")) -> ()  [unwired: 13 in, 1 out]
      }
      frame "Data: Insert After" {
        n144 = Decimal String To Number(string=w271) -> (number=w270:i32)  [unwired: 2 in, 1 out]
        n145 = Increment(x=w270) -> (x+1=w269:i32)
        n146 = in-place {
          in-place-border: w269 -> [w276]
          n147 = in-place-cluster #7(w272) -> ("Steps"=w279:T7[])
          n148 = call "Alter Motor Profile V2.vi"("Action"=enum16{"Add", "Insert", "Modify", "Delete"}."Insert", "Step"=w276, "Steps in"=w279) -> ("Steps out"=w278:T7[])  [unwired: 8 in]
          n149 = in-place-cluster #7("Steps"=w278) -> (w274:T13)
        }
        n150 = call "Enqueue Multiple States.vi"("queue in"=w268, "State(s) at Back"="UI: Display Process" ("State(s) at Back (\"\")")) -> ()  [unwired: 13 in, 1 out]
      }
      frame "Data: Modify" {
        n151 = Decimal String To Number(string=w282) -> (number=w281:i32)  [unwired: 2 in, 1 out]
        n152 = in-place {
          in-place-border: w281 -> [w287]
          n153 = in-place-cluster #8(w283) -> ("Steps"=w290:T7[])
          n154 = call "Alter Motor Profile V2.vi"("Action"=enum16{"Add", "Insert", "Modify", "Delete"}."Modify", "Step"=w287, "Steps in"=w290) -> ("Steps out"=w289:T7[])  [unwired: 8 in]
          n155 = in-place-cluster #8("Steps"=w289) -> (w285:T13)
        }
        n156 = call "Enqueue Multiple States.vi"("queue in"=w280, "State(s) at Back"="UI: Display Process" ("State(s) at Back (\"\")")) -> ()  [unwired: 13 in, 1 out]
      }
      frame "Data: Delete" {
        n157 = Decimal String To Number(string=w293) -> (number=w292:i32)  [unwired: 2 in, 1 out]
        n158 = in-place {
          in-place-border: w292 -> [w298]
          n159 = in-place-cluster #9(w294) -> ("Steps"=w301:T7[])
          n160 = call "Alter Motor Profile V2.vi"("Action"=enum16{"Add", "Insert", "Modify", "Delete"}."Delete", "Step"=w298, "Steps in"=w301) -> ("Steps out"=w300:T7[])  [unwired: 8 in]
          n161 = in-place-cluster #9("Steps"=w300) -> (w296:T13)
        }
        n162 = call "Enqueue Multiple States.vi"("queue in"=w291, "State(s) at Back"="UI: Display Process" ("State(s) at Back (\"\")")) -> ()  [unwired: 13 in, 1 out]
      }
      frame "Data: Clear Profile" {
        n163 = call "Display Message to User"() -> ("OK"=w305:bool)  [unwired: 10 in, 1 out]
        n164 = case shown="True" w305 {
          tunnel: w304 -> [w308 w312]
          tunnel: [w308 w311] -> w303
          frame False {
          }
          frame True {
            n165 = Bundle By Name(cluster=w312, "Steps"=T7[] []) -> (w311:T13)
            n166 = property on="Table" class="Tbl (strict)"("Index Values"=T9 {"Row"=0, "Column"=0}) -> ()  [unwired: 2 in, 2 out]
          }
        }
        n167 = call "Enqueue Multiple States.vi"("queue in"=w302, "State(s) at Back"="UI: Display Process" ("State(s) at Back (\"\")")) -> ()  [unwired: 13 in, 1 out]
      }
      frame "Data: Save Process" {
        n168 = local read "Process Name"() -> (w319:string)
        n169 = Unbundle By Name(w314) -> ("Config"=w315:T12)
        n170 = call <vilib>:"Get Section Names.vi"("refnum"=w315) -> ("error out"=w318:errorcluster, "section names"=w316:string[])  [unwired: 8 in, 1 out]
        n171 = Unbundle By Name(w314) -> ("Steps"=w327:T7[])
        n172 = Search 1D Array(1D array=w316, element=w319) -> (index of element=w317:i32)  [unwired: 1 in]
        n173 = Bundle("Steps"=w327, "Activation Type"="Activation Type", "N"="N") -> (w324:T10)  [unwired: 1 in]
        n174 = case shown="0, Default" w317 {
          tunnel: w318 -> [w348 w349]
          tunnel: [w347 w349] -> _
          tunnel: [w346 TRUE ("Overwrite")] -> w313
          frame 0, Default {
            n175 = call "Overwrite?"("error in (no error)"=w348) -> ("error out"=w347:errorcluster, "Overwrite"=w346:bool)  [unwired: 9 in]
          }
          frame -1 {
          }
        }
        n176 = Flatten To String(anything=w324) -> (data string=w322:string)  [unwired: 3 in, 2 out]
        n177 = case shown="True" w313 {
          tunnel: w323 -> [w328 w334]
          tunnel: w322 -> [_ w333]
          tunnel: [w328 w332] -> w321
          tunnel: [w329 w331] -> w320
          tunnel: w314 -> [w329 w330]
          frame False {
          }
          frame True {
            n178 = in-place {
              in-place-border: w334 -> [w343]
              in-place-border: w333 -> [w342]
              in-place-border: [w336] -> w332
              n179 = in-place-cluster #10(w330) -> ("Config"=w345:T12)
              n180 = local read "Process Name"() -> (w335:string)
              n181 = call-poly <vilib>:"Write Key.vi"("section"=w335, "error in (no error)"=w343, "value"=w342, "key"="data", "refnum"=w345) -> ("error out"=w340:errorcluster, "refnum out"=w341:T12)  [unwired: 4 in, 1 out]
              n182 = call <vilib>:"Close Config Data.vi"("error in (no error)"=w340, "refnum"=w341) -> ("error out"=w338:errorcluster, "file path"=w339:path)  [unwired: 8 in]
              n183 = call <vilib>:"Open Config Data.vi"("error in (no error)"=w338, "configuration file path"=w339) -> ("error out"=w336:errorcluster, "refnum"=w337:T12)  [unwired: 7 in, 1 out]
              n184 = in-place-cluster #10("Config"=w337) -> (w331:T13)
            }
          }
        }
      }
      frame "Data: Load Process" {
        n185 = local read "Process Name"() -> (w366:string)
        n186 = Unbundle By Name(w351) -> ("Config"=w364:T12)
        n187 = call-poly <vilib>:"Read Key.vi"("section"=w366, "error in (no error)"=w365, "key"="data", "refnum"=w364) -> ("error out"=w361:errorcluster, "value"=w362:string, "found?"=w355:bool)  [unwired: 4 in, 1 out]
        n188 = case shown="False" w355 {
          tunnel: w362 -> [_ w379]
          tunnel: w361 -> [w371 w378]
          tunnel: [w371 w377] -> w360
          tunnel: [w368 w374] -> w358
          tunnel: [w367 w373] -> w357
          tunnel: [w369 w372] -> w353
          tunnel: w351 -> [w370 _]
          frame False {
            n189 = Unbundle By Name(w370) -> ("Steps"=w369:T7[])
            n190 = property on="Activation Type" class="RadioBtnsControl (strict)"() -> ("Value"=w368:enum32{"Hotkey", "Automatic"})  [unwired: 2 in, 2 out]
            n191 = property on="N" class="DigNum (strict)"() -> ("Value"=w367:i32)  [unwired: 2 in, 2 out]
          }
          frame True {
            n192 = Unflatten From String(type=T10 {"Steps"=[], "Activation Type"=enum."Hotkey", "N"=0} ("cluster"), binary string=w379, error in (no error)=w378) -> (value=w376:T10, error out=w377:errorcluster)  [unwired: 2 in, 1 out]
            n193 = Unbundle By Name(w376) -> ("Steps"=w372:T7[], "Activation Type"=w374:enum32{"Hotkey", "Automatic"}, "N"=w373:i32)
          }
        }
        n194 = call-poly <userlib>:"MGI Gray if.vi"("Boolean"=w355) -> ("Disabled"=w356:T2)
        n195 = property on="Restore" class="Bool"("DisabledEnum"=w356) -> ()  [unwired: 2 in, 2 out]
        n196 = property on="Activation Type" class="RadioBtnsControl (strict)"("Val(Sgnl)"=w358) -> ()  [unwired: 2 in, 2 out]
        n197 = property on="N" class="DigNum (strict)"("Val(Sgnl)"=w357) -> ()  [unwired: 2 in, 2 out]
        n198 = call "Enqueue Multiple States.vi"("queue in"=w354, "State(s) at Back"="UI: Display Process" ("State(s) at Back (\"\")")) -> ()  [unwired: 13 in, 1 out]
        n199 = Bundle By Name(cluster=w351, "Steps"=w353) -> (w352:T13)
      }
      frame "Data: Delete Process" {
        n200 = call "Perm Delete?"("error in (no error)"=w382) -> ("error out"=w383:errorcluster, "Delete"=w384:bool)  [unwired: 9 in]
        n201 = case shown="True" w384 {
          tunnel: w383 -> [w385 w392]
          tunnel: [w385 w387] -> w381
          tunnel: w380 -> [_ w391]
          frame False {
          }
          frame True {
            n202 = local read "Process Name"() -> (w389:string)
            n203 = Unbundle By Name(w391) -> ("Config"=w390:T12)
            n204 = call <vilib>:"Remove Section.vi"("section"=w389, "error in (no error)"=w392, "refnum"=w390) -> ("error out"=w388:errorcluster)  [unwired: 6 in, 2 out]
            n205 = property on="Process Name" class="CmbBox"(error in=w388, "Val(Sgnl)"="") -> (error out=w387:errorcluster)  [unwired: 1 in, 1 out]
          }
        }
      }
      frame "Data: Cleanup" {
        # "Cleanup any data and references, here.\n(this is called automatically, by the Macro: Exit)"
        n206 = Unbundle By Name(w400) -> ("Core.Current VI Reference"=w399:refnum<vi>, "Keyboard"=w393:refnum<k1>)
        n207 = Close Reference(reference=w399, error in (no error)=w397) -> (error out=w394:errorcluster)
        n208 = call-poly <vilib>:"Close Input Device.vi"("error in (no error)"=w394, "device ID"=w393) -> ("error out"=w395:errorcluster)  [unwired: 8 in]
        n209 = invoke class="VI" method="Default Vals.Reinit All"(error in=w395) -> (error out=w398:errorcluster)  [unwired: 2 in, 2 out]
        n210 = call "Enqueue Multiple States.vi"("queue in"=w396) -> ()  [unwired: 14 in, 1 out]
      }
      frame "---------- UI ----------" {
        # "Do not put any code in this frame.\n(It is a separator no-op. You can make a copy of this frame to create a new UI frame)"
        n211 = call "Enqueue Multiple States.vi"("queue in"=w401) -> ()  [unwired: 14 in, 1 out]
      }
      frame "UI: Initialize" {
        w411 = T2."Disabled and Grayed Out" ("Disabled")
        # "Initialize the User Interface, here.\n(this is called automatically, by the Macro: Init)"
        n212 = property on="Start/Stop" class="Bool (strict)"("DisabledEnum"=w411) -> ()  [unwired: 2 in, 2 out]
        n213 = property on="Restore" class="Bool"("DisabledEnum"=w411) -> ()  [unwired: 2 in, 2 out]
        n214 = property on="Save" class="Bool"("DisabledEnum"=w411) -> ()  [unwired: 2 in, 2 out]
        n215 = call "Hotkey FGV.vi"("error in (no error)"=w409) -> ("error out"=w408:errorcluster, "Hotkey String out"=→"Application Hotkey":string, "Hotkey out"=w404:T14)  [unwired: 8 in]
        n216 = Bundle By Name(cluster=w406, "Hotkey"=w404) -> (w405:T13)
        n217 = call "Enqueue Multiple States.vi"("queue in"=w410) -> ()  [unwired: 14 in, 1 out]
      }
      frame "UI: Cursor Set" {
        # "Argument"
        # "Set and Unset Cursor Busy.\n(Usage: \"UI: Cursor Set >> Busy|Idle\")"
        n218 = case shown="\"Idle\", Default" w413 {
          tunnel: w415 -> [w418 w420]
          tunnel: [w417 w419] -> w414
          frame "Idle", Default {
            n219 = call <vilib>:"Unset Busy.vi"("error in (no error)"=w418) -> ("error out"=w417:errorcluster)  [unwired: 10 in]
          }
          frame "Busy" {
            n220 = call <vilib>:"Set Busy.vi"("error in (no error)"=w420) -> ("error out"=w419:errorcluster)  [unwired: 9 in, 1 out]
          }
        }
        n221 = call "Enqueue Multiple States.vi"("queue in"=w412) -> ()  [unwired: 14 in, 1 out]
      }
      frame "UI: Front Panel State" {
        # "Argument"
        # "Set Front Panel Open or Closed\n(Usage: \"UI: Front Panel State >> Open|Close\")"
        n222 = Unbundle By Name(w424) -> ("Core.Current VI Reference"=w423:refnum<vi>)
        n223 = case shown="\"Hidden\", \"Hide\"" w422 {
          tunnel: w426 -> [w432 w447 w458 w471 w484]
          tunnel: [w434 w448 w460 w473 w486] -> w425
          tunnel: w423 -> [w433 w445 w459 w472 w485]
          frame "Open", "Standard", Default {
            w427 = T5."Standard" ("State")
            n224 = property class="VI"(reference=w433, error in=w432) -> (reference out=w430:refnum<vi>, error out=w431:errorcluster, "FP.State"=w429:T5)
            n225 = Not Equal?(x=w429, y=w427) -> (x != y?=w428:bool)
            n226 = case shown="False" w428 {
              tunnel: [w438 w440] -> w434
              tunnel: w431 -> [w437 w440]
              tunnel: w430 -> [w436 _]
              tunnel: w427 -> [w435 _]
              frame True {
                n227 = invoke class="VI" method="FP.Open"(reference=w436, error in=w437, "Activate"=TRUE, "State"=w435) -> (error out=w438:errorcluster)  [unwired: 1 in, 4 out]
              }
              frame False {
              }
            }
          }
          frame "Close", "Closed" {
            n228 = property class="VI"(reference=w445, error in=w447) -> (reference out=w444:refnum<vi>, error out=w446:errorcluster, "FP.State"=w442:T5)
            n229 = Not Equal?(x=w442, y=T5."Closed" ("Front Panel Window:State")) -> (x != y?=w441:bool)
            n230 = case shown="True" w441 {
              tunnel: [w449 w452] -> w448
              tunnel: w446 -> [w449 w451]
              tunnel: w444 -> [_ w450]
              frame False {
              }
              frame True {
                n231 = invoke class="VI" method="FP.Close"(reference=w450, error in=w451) -> (error out=w452:errorcluster)  [unwired: 1 in, 2 out]
              }
            }
          }
          frame "Hidden", "Hide" {
            w453 = T5."Hidden" ("State")
            n232 = property class="VI"(reference=w459, error in=w458) -> (reference out=w456:refnum<vi>, error out=w457:errorcluster, "FP.State"=w455:T5)
            n233 = Not Equal?(x=w455, y=w453) -> (x != y?=w454:bool)
            n234 = case shown="True" w454 {
              tunnel: [w464 w465] -> w460
              tunnel: w457 -> [w463 w465]
              tunnel: w456 -> [w462 _]
              tunnel: w453 -> [w461 _]
              frame True {
                n235 = invoke class="VI" method="FP.Open"(reference=w462, error in=w463, "State"=w461) -> (error out=w464:errorcluster)  [unwired: 2 in, 4 out]
              }
              frame False {
              }
            }
          }
          frame "Minimize", "Minimized" {
            w466 = T5."Minimized" ("State")
            n236 = property class="VI"(reference=w472, error in=w471) -> (reference out=w469:refnum<vi>, error out=w470:errorcluster, "FP.State"=w468:T5)
            n237 = Not Equal?(x=w468, y=w466) -> (x != y?=w467:bool)
            n238 = case shown="True" w467 {
              tunnel: [w477 w478] -> w473
              tunnel: w470 -> [w476 w478]
              tunnel: w469 -> [w475 _]
              tunnel: w466 -> [w474 _]
              frame True {
                n239 = invoke class="VI" method="FP.Open"(reference=w475, error in=w476, "State"=w474) -> (error out=w477:errorcluster)  [unwired: 2 in, 4 out]
              }
              frame False {
              }
            }
          }
          frame "Maximize", "Maximized" {
            w479 = T5."Maximized" ("State")
            n240 = property class="VI"(reference=w485, error in=w484) -> (reference out=w482:refnum<vi>, error out=w483:errorcluster, "FP.State"=w481:T5)
            n241 = Not Equal?(x=w481, y=w479) -> (x != y?=w480:bool)
            n242 = case shown="True" w480 {
              tunnel: [w490 w491] -> w486
              tunnel: w483 -> [w489 w491]
              tunnel: w482 -> [w488 _]
              tunnel: w479 -> [w487 _]
              frame True {
                n243 = invoke class="VI" method="FP.Open"(reference=w488, error in=w489, "State"=w487) -> (error out=w490:errorcluster)  [unwired: 2 in, 4 out]
              }
              frame False {
              }
            }
          }
        }
        n244 = call "Enqueue Multiple States.vi"("queue in"=w421) -> ()  [unwired: 14 in, 1 out]
      }
      frame "UI: Populate Processes" {
        n245 = Unbundle By Name(w496) -> ("Config"=w493:T12)
        n246 = call <vilib>:"Get Section Names.vi"("error in (no error)"=w495, "refnum"=w493) -> ("error out"=w494:errorcluster, "section names"=w492:string[])  [unwired: 7 in, 1 out]
        n247 = property on="Process Name" class="CmbBox"("Strings[]"=w492) -> ()  [unwired: 2 in, 2 out]
      }
      frame "UI: Display Process" {
        n248 = Unbundle By Name(w510) -> ("Steps"=w506:T7[])
        n249 = local read "Process Name"() -> (w504:string)
        n250 = Empty Array?(array=w506) -> (empty?=w505:bool)
        n251 = Empty String/Path?(string/path=w504) -> (empty?=w503:bool)
        n252 = Not(x=w503) -> (.not. x?=w502:bool)
        n253 = Not(x=w505) -> (.not. x?=w499:bool)
        n254 = And(x=w502, y=w499) -> (x .and. y?=w501:bool)
        n255 = call-poly <userlib>:"MGI Gray if.vi"("Boolean"=w501) -> ("Disabled"=w500:T2)
        n256 = call-poly <userlib>:"MGI Gray if.vi"("Boolean"=w499) -> ("Disabled"=w498:T2)
        n257 = call "Display Data to Table.vi"("error in (no error)"=w508, "Test Data In"=w506) -> ("error out"=w507:errorcluster, "Array"=→"Table":string[][])  [unwired: 8 in]
        n258 = property on="Save" class="Bool"("DisabledEnum"=w500) -> ()  [unwired: 2 in, 2 out]
        n259 = property on="Start/Stop" class="Bool (strict)"("DisabledEnum"=w498) -> ()  [unwired: 2 in, 2 out]
        n260 = call "Enqueue Multiple States.vi"("queue in"=w497) -> ()  [unwired: 14 in, 1 out]
      }
      frame "UI: Refs" {
        n261 = Unbundle By Name(w514) -> ("Refs"=w512:refnum<vi>[])
        n262 = case shown="\"Disable\", Default" w515 {
          tunnel: [FALSE TRUE] -> _
          tunnel: [T2."Disabled and Grayed Out" ("Enum Out") T2."Enabled" ("Disabled")] -> w511
          frame "Disable", Default {
          }
          frame "Enable" {
          }
        }
        n263 = for {
          tunnel: w512 -> [w517] mode=indexing
          tunnel: w511 -> [w516]
          n264 = property class="Ctl"(reference=w517, "DisabledEnum"=w516) -> ()  [unwired: 1 in, 2 out]
        }
      }
      frame "UI: Wait" {
        n265 = call "Timer FGV.vi"("Mode"=FGV_Actions."Read", "error in (no error)"=w526) -> ("error out"=w529:errorcluster, "Expired?"=w527:bool)  [unwired: 7 in, 1 out]
        n266 = Select(t="Macro: Process >> Step", s=w527, f="UI: Wait") -> (s? t:f=w523:string)
        n267 = call "Enqueue Multiple States.vi"("queue in"=w522, "State(s) at Back"=w523) -> ()  [unwired: 13 in, 1 out]
      }
      frame "UI: Listen" {
        n268 = Unbundle By Name(w535) -> ("Hotkey"=w531:T14, "Keyboard"=w544:refnum<k1>)
        n269 = call "Stall Data Flow.vim"("value in"=w544, "milliseconds to wait"=u32 1) -> ("value out"=w539:refnum<k1>)  [unwired: 1 out]
        n270 = call-poly <vilib>:"Acquire Input Data.vi"("device ID"=w539, "error in (no error)"=w537) -> ("keys pressed"=w543:T14, "error out"=w536:errorcluster)  [unwired: 15 in, 1 out]
        n271 = Sort 1D Array(array=w543) -> (sorted array=w542:T14)
        n272 = Equal?(x=w531, y=w542) -> (x = y?=w541:bool)
        n273 = Select(t="Macro: Process >> Start", s=w541, f="UI: Listen" ("string")) -> (s? t:f=w534:string)
        n274 = call "Enqueue Multiple States.vi"("queue in"=w532, "State(s) at Back"=w534) -> ()  [unwired: 13 in, 1 out]
      }
      frame "---------- Macro ----------" {
        # "Do not put any code in this frame.\n(It is a separator no-op. You can make a copy of this frame to create a new Macro frame)"
        n275 = call "Enqueue Multiple States.vi"("queue in"=w545) -> ()  [unwired: 14 in, 1 out]
      }
      frame "Macro: Initialize" {
        w549 = "Data: Initialize\nInitialize Core Data\nUI: Refs >> Enable\nUI: Initialize\nData: Open Config\nUI: Populate Processes\nUI: Front Panel State >> Open"  # Data: Initialize Initialize Core Data UI: Refs >> Enable UI: Initialize Data: Open Config UI: Populate Processes UI: Front Panel State >> Open
        # "Initialization Macro\n(This is called once, when the VI starts)"
        n276 = call "Enqueue Multiple States.vi"("State(s) at Front"=w549, "queue in"=w548) -> ()  [unwired: 13 in, 1 out]
      }
      frame "Macro: Process" {
        n277 = case shown="\"Start\", Default" w556 {
          tunnel: w552 -> [w561 w565 w570 w585 w589]
          tunnel: [w560 w564 w568 w583 w589] -> w555
          tunnel: ["Process: Perform Step" "Process: Perform Step" w566 w581 w588] -> w554
          frame "Start", Default {
            w558 = 0 ("Step")
            n278 = Bundle By Name(cluster=w561, "Step"=w558, "n"=w558) -> (w560:T13)
          }
          frame "Repeat" {
            n279 = Bundle By Name(cluster=w565, "Step"=0) -> (w564:T13)
          }
          frame "Step" {
            n280 = Unbundle By Name(w570) -> ("Step"=w575:i32, "Steps"=w573:T7[])
            n281 = Array Size(array=w573) -> (size(s)=w574:i32)
            n282 = Increment(x=w575) -> (x+1=w569:i32)
            n283 = Greater Or Equal?(x=w569, y=w574) -> (x >= y?=w572:bool)
            n284 = Select(t="Macro: Process >> Complete", s=w572, f="Process: Perform Step") -> (s? t:f=w566:string)
            n285 = Bundle By Name(cluster=w570, "Step"=w569) -> (w568:T13)
          }
          frame "Complete" {
            n286 = Unbundle By Name(w585) -> ("n"=w587:i32)
            n287 = Increment(x=w587) -> (x+1=w584:i32)
            n288 = local read "N"() -> (w580:i32)
            n289 = Greater?(x=w584, y=w580) -> (0:w578:bool)
            n290 = Not Equal?(x=w580, y=-1) -> (x != y?=w577:bool)
            n291 = And(x=w578, y=w577) -> (x .and. y?=w576:bool)
            n292 = Select(t="Macro: Process >> End", s=w576, f="Macro: Process >> Repeat") -> (s? t:f=w581:string)
            n293 = Bundle By Name(cluster=w585, "n"=w584) -> (w583:T13)
          }
          frame "End" {
            n294 = local read "Activation Type"() -> (w592:enum32{"Hotkey", "Automatic"})
            n295 = Equal?(x=w592, y=enum32{"Hotkey", "Automatic"}."Hotkey") -> (x = y?=w590:bool)
            n296 = case shown="False" w590 {
              tunnel: [_ "UI: Listen"] -> w588
              frame False {
                n297 = property on="Start/Stop" class="Bool (strict)"("Val(Sgnl)"=FALSE ("Value (Signaling)")) -> ()  [unwired: 2 in, 2 out]
              }
              frame True {
              }
            }
          }
        }
        n298 = call "Enqueue Multiple States.vi"("queue in"=w553, "State(s) at Back"=w554) -> ()  [unwired: 13 in, 1 out]
      }
      frame "Macro: Exit" {
        # "Exit Macro\n(This is called once, when the VI exits)"
        n299 = Unbundle By Name(w602) -> ("Core.Close Panel on Exit?"=w601:bool)
        n300 = property on="Table" class="Tbl (strict)"("Index Values"=T9 {"Row"=0, "Column"=0}) -> ()  [unwired: 2 in, 2 out]
        n301 = Select(t="UI: Front Panel State >> Close", s=w601, f="") -> (s? t:f=w596:string)
        n302 = call "Enqueue Multiple States.vi"("State(s) at Front"=w596, "queue in"=w597, "State(s) at Back"="Data: Cleanup\nExit") -> ()  [unwired: 12 in, 1 out]
      }
      frame "---------- Process ----------" {
        n303 = call "Enqueue Multiple States.vi"("queue in"=w604) -> ()  [unwired: 14 in, 1 out]
      }
      frame "Process: Perform Step" {
        n304 = Unbundle By Name(w624) -> ("Steps"=w623:T7[], "Step"=w622:i32)
        n305 = Index Array(array=w623, index=w622) -> (element=w621:T7)
        n306 = Unbundle By Name(w621) -> ("Repeat"=w611:i32, "Type"=w620:T8, "Coords"=w619:cluster{"x":i32, "y":i32}, "Delay"=w618:i32, "Key"=w617:u8, "RClick?"=w613:bool)
        n307 = Increment(x=w611) -> (x+1=w610:i32)
        n308 = Equal To 0?(x=w610) -> (x = 0?=w612:bool)
        n309 = Select(t=2147483647, s=w612, f=w610) -> (s? t:f=w609:i32)
        n310 = for {
          N: w609 -> [_]
          tunnel: w620 -> [w632]
          tunnel: w619 -> [w631]
          tunnel: w618 -> [w630]
          tunnel: w617 -> [w629]
          tunnel: [w626] -> w614
          tunnel: w613 -> [w625]
          shift-right: [w627] -> w615
          shift-left: w616 -> [w628]
          n311 = case shown="\"Mouse Click\"" w632 {
            tunnel: w631 -> [w639 _ _ _ _ _ _ _]
            tunnel: w630 -> [w636 w645 w655 w659 w664 w670 w675 w681]
            tunnel: w629 -> [_ _ w650 _ _ w669 w674 _]
            tunnel: w628 -> [w640 w648 w657 w662 w667 w672 w677 w684]
            tunnel: [w637 w647 w656 w661 w666 w671 w676 w683] -> w627
            tunnel: ["Macro: Process >> Step" "Macro: Process >> Step" "Macro: Process >> Step" "Macro: Process >> Step" "Macro: Process >> Step" "Macro: Process >> Step" "Macro: Process >> Step" "UI: Wait"] -> w626
            tunnel: w625 -> [_ w646 _ w660 w665 _ _ _]
            frame "Mouse Move", Default {
              n312 = Unbundle By Name(w639) -> ("x"=w635:i32, "y"=w634:i32)
              n313 = call "Mouse Move.vi"("error in (no error)"=w640, "y"=w634, "x"=w635) -> ("error out"=w638:errorcluster)  [unwired: 8 in]
              n314 = call "Stall Data Flow.vim"("value in"=w638, "milliseconds to wait"=w636) -> ("value out"=w637:errorcluster)  [unwired: 1 out]
            }
            frame "Mouse Click" {
              n315 = Quotient & Remainder(x=w645, y=2) -> (x-y*floor(x/y)=w643:i32, floor(x/y)=w641:i32)
              n316 = Add(x=w643, y=w641) -> (x+y=w642:i32)
              n317 = call "Mouse Click.vi"("error in (no error)"=w648, "ms wait after up (10)"=w642, "ms wait after down (10)"=w641, "Right Click? (F)"=w646) -> ("error out"=w647:errorcluster)  [unwired: 7 in]
            }
            frame "Key Press" {
              n318 = Quotient & Remainder(x=w655, y=2) -> (x-y*floor(x/y)=w653:i32, floor(x/y)=w651:i32)
              n319 = Add(x=w653, y=w651) -> (x+y=w652:i32)
              n320 = call "Key Press.vi"("error in (no error)"=w657, "ms wait after up (20)"=w652, "ms wait after down (80)"=w651, "Virtual Key"=w650) -> ("error out"=w656:errorcluster)  [unwired: 7 in]
            }
            frame "Mouse Down" {
              n321 = call "Mouse Down.vi"("error in (no error)"=w662, "Delay in ms (10)"=w659, "Right Click? (F)"=w660) -> ("error out"=w661:errorcluster)  [unwired: 8 in]
            }
            frame "Mouse Up" {
              n322 = call "Mouse Up.vi"("error in (no error)"=w667, "Delay in ms (10)"=w664, "Right Click? (F)"=w665) -> ("error out"=w666:errorcluster)  [unwired: 8 in]
            }
            frame "Key Down" {
              n323 = call "Key Down.vi"("error in (no error)"=w672, "delay in ms (80)"=w670, "Virtual Key"=w669) -> ("error out"=w671:errorcluster)  [unwired: 8 in]
            }
            frame "Key Up" {
              n324 = call "Key Up.vi"("error in (no error)"=w677, "delay in ms (20)"=w675, "Virtual Key"=w674) -> ("error out"=w676:errorcluster)  [unwired: 8 in]
            }
            frame "Wait" {
              n325 = Divide(x=w681, y=1000) -> (x/y=w679:dbl)
              n326 = call "Timer FGV.vi"("Mode"=FGV_Actions."Write", "error in (no error)"=w684, "Timer Value (s)"=w679) -> ("error out"=w683:errorcluster)  [unwired: 6 in, 2 out]
            }
          }
        }
        n327 = call "Enqueue Multiple States.vi"("queue in"=w608, "State(s) at Back"=w614) -> ()  [unwired: 13 in, 1 out]
      }
    }
  }
  n328 = Merge Errors(w9, w8) -> (w10:errorcluster)
  n329 = Release Queue(queue=w11, error in (no error)=w10) -> (error out=→"error out":errorcluster)  [unwired: 1 in, 2 out]
